vi "HypervisorFinalWriteAndClose.vi"(8 "ErrorIn":errorcluster, 11 "QIn":refnum<queue>) -> (0 "ErrorOut":errorcluster)   [LabVIEW 2018]
doc: "This VI calls for the final logging of any remaining events in the Hypervisor loop and then closes the Queue.\n\n\nCopyright © 2011 Epimedia, Inc. All Rights Reserved.\n\nThe Epimedia Application Library is Copyright © 2009-2011 Epimedia, Inc. \nAll Rights Reserved. Used under license."
uses:
  HyperVisor.ctl
panel:
  # "Copyright © 2011 Epimedia, Inc. All Rights Reserved.\n\nThe Epimedia Application Library is Copyright © 2009-2011 Epimedia, Inc. \nAll Rights Reserved. Used under license."
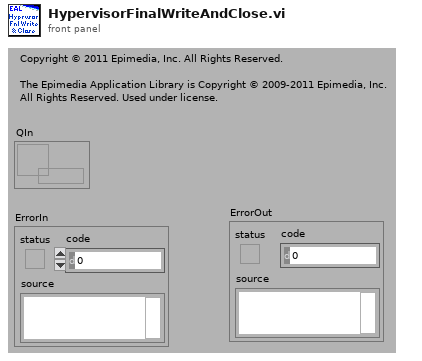
[diagram p1: front panel]
types:
  T1 = typedef "HyperVisor.ctl" = cluster{"TimeOut":dbl, string, "Data":variant, "StopHpvsr":bool}
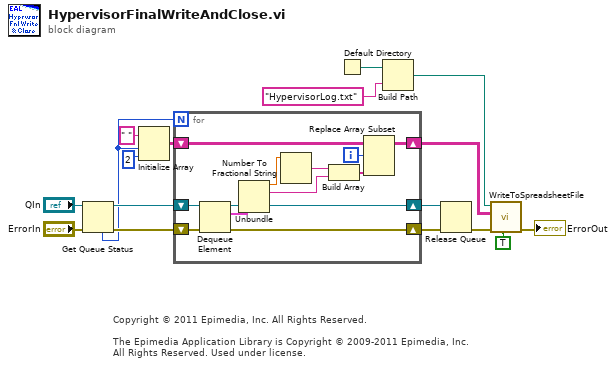
[diagram p0: block diagram]
diagram:
  # "Copyright © 2011 Epimedia, Inc. All Rights Reserved.\n\nThe Epimedia Application Library is Copyright © 2009-2011 Epimedia, Inc. \nAll Rights Reserved. Used under license."
  n1 = Get Queue Status(queue="QIn", error in (no error)="ErrorIn") -> (queue out=w9:refnum<queue>, error out=w7:errorcluster, # elements in queue=w2:i32)  [unwired: 1 in, 5 out]
  n2 = Initialize Array(" ", w2, 2 ("dimension size")) -> (w14:string[][])
  n3 = for {
    N: w2 -> [_]
    shift-right: [w23] -> w13
    shift-left: w14 -> [w29]
    shift-right: [w22] -> w6
    shift-left: w9 -> [w20]
    shift-right: [w18] -> w5
    shift-left: w7 -> [w21]
    i -> [w24]
    n4 = Dequeue Element(queue=w20, error in (no error)=w21) -> (queue out=w22:refnum<queue>, element=w19:T1, error out=w18:errorcluster)  [unwired: 2 out]
    n5 = Unbundle(w19) -> ("TimeOut"=w28:dbl, w27:string)  [unwired: 2 out]
    n6 = Number To Fractional String(number=w28) -> (F-format string=w26:string)  [unwired: 1 in, 2 out]
    n7 = Build Array(w26, w27) -> (w25:string[])
    n8 = Replace Array Subset(array=w29, new element=w25, index (row)=w24) -> (w23:string[][])  [unwired: 1 in]
  }
  n9 = Default Directory() -> (w1:path)
  n10 = Build Path(base path=w1, name or relative path="HypervisorLog.txt") -> (appended path=w11:path)
  n11 = Release Queue(queue=w6, error in (no error)=w5) -> (error out=w4:errorcluster)  [unwired: 1 in, 2 out]
  n12 = call "WriteToSpreadsheetFile.vi"("Append?(NewFile:F)"=TRUE ("append to file? (new file:F)"), "ErrorIn"=w4, "2D-Data"=w13, "FilePath(DialogIfEmpty)"=w11) -> ("ErrorOut"=→"ErrorOut":errorcluster)  [unwired: 4 in, 3 out]
